vi "VI Tree.vi"   [LabVIEW 2012, in "Phidget Light Sensor.lvlib"]
doc: "${LightSensor:VITreeHeader}"
uses:
  <instrlib>/Phidgets/Phidget Light Sensor/Phidget Light Sensor.lvlib
  <instrlib>/Phidgets/Phidget Light Sensor/Public/LightSensorStart.vi
  <instrlib>/Phidgets/Phidget Light Sensor/Public/LightSensorOpen.vi
  <instrlib>/Phidgets/Phidget Light Sensor/Public/LightSensorClose.vi
panel:
  # "(c) 2015 Phidgets Inc..  ALL RIGHTS RESERVED."
  # "SEE DIAGRAM\nFOR VI TREE."
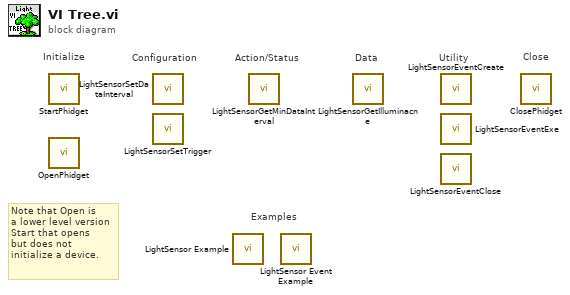
[diagram p0: block diagram]
diagram:
  # "Note that Open is\na lower level version\nStart that opens\nbut does not \ninitialize a device."
  # "Examples"
  # "Configuration"
  # "Utility"
  # "Data"
  # "Action/Status"
  # "Close"
  # "Initialize"
  n1 = call-poly <instrlib>:"StartPhidget.vi"() -> ()  [unwired: 12 in, 4 out]
  n2 = call-poly <instrlib>:"OpenPhidget.vi"() -> ()  [unwired: 8 in, 4 out]
  n3 = call <instrlib>:"LightSensorSetDataInterval.vi"() -> ()  [unwired: 9 in, 2 out]
  n4 = call <instrlib>:"LightSensorSetTrigger.vi"() -> ()  [unwired: 9 in, 2 out]
  n5 = call <instrlib>:"LightSensor Example.vi"() -> ()  [unwired: 12 in]
  n6 = call <instrlib>:"LightSensorGetMinDataInterval.vi"() -> ()  [unwired: 8 in, 3 out]
  n7 = call <instrlib>:"LightSensor Event Example.vi"() -> ()  [unwired: 12 in]
  n8 = call <instrlib>:"LightSensorGetIlluminacne.vi"() -> ()  [unwired: 8 in, 3 out]
  n9 = call <instrlib>:"LightSensorEventCreate.vi"() -> ()  [unwired: 9 in, 3 out]
  n10 = call <instrlib>:"LightSensorEventExe.vi"() -> ()  [unwired: 5 in, 7 out]
  n11 = call <instrlib>:"LightSensorEventClose.vi"() -> ()  [unwired: 10 in, 2 out]
  n12 = call-poly <instrlib>:"ClosePhidget.vi"() -> ()  [unwired: 11 in, 1 out]
